vi "1B_BFG Ramp Data.vi"(7 "array":dbl[][](array[numeric])=array2400x3[7200 elements]) -> (8 "Threshold Values":u16[](array[numeric]))   [LabVIEW 2010]
panel:
  # "•\tBattery 75% Voltage Threshold, No Load: 3.950V\n•\tBattery 75% Voltage Threshold, Stimulation On: 3.925V\n•\tBattery 50% Voltage Threshold, No Load: 3.850V\n•\tBattery 50% Voltage Threshold, Stimulation On: 3.825V\n•\tBattery 25% Voltage Threshold, No Load: 3.780V\n•\tBattery 25% Voltage Threshold, Stimulation On: 3.755V\n•\tBattery Warning Voltage Threshold, No Load: 3.740V\n•\tBattery Warning Voltage Threshold, Stimulation On: 3.715V\n•\tBattery Critical Voltage Threshold, No Load: 3.720V\n•\tBattery Critical Voltage Threshold, Stimulation On: 3.695V\n•\tMinimum Safe Stimulating Voltage, No Load: 3.700V\n•\tMinimum Safe Stimulation Voltage, Stimulation On: 3.675V\n•\tBattery Cut-off Voltage Threshold:  2.850V"
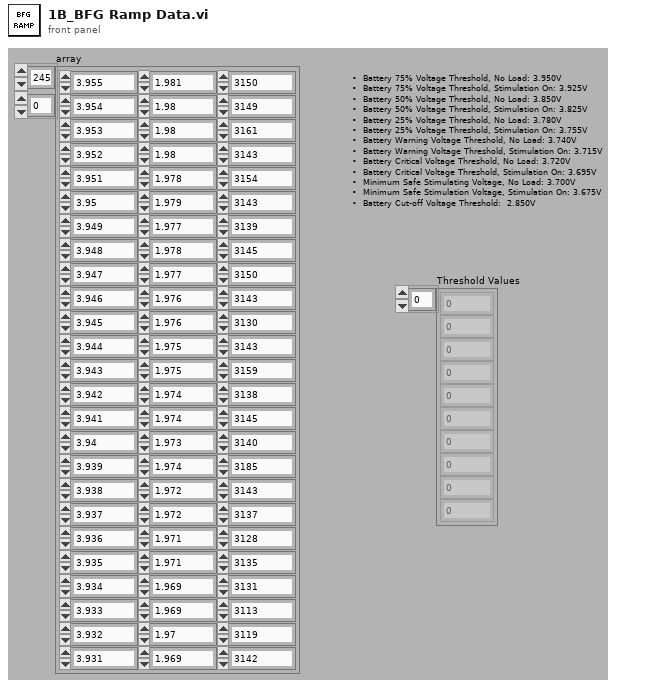
[diagram p1: front panel]
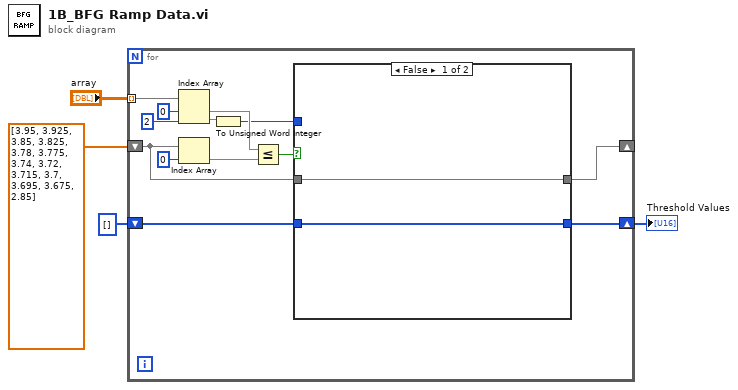
[diagram p0: block diagram]
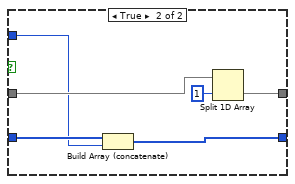
[diagram p2: hidden frame]
diagram:
  n1 = for {
    tunnel: "array" -> [w16] mode=indexing
    shift-right: [w6] -> _
    shift-left: dbl[] [3.95, 3.925, 3.85, 3.825, 3.78, 3.775, 3.74, 3.72, 3.715, 3.7, 3.695, 3.675, 2.85] -> [w7]
    shift-right: [w5] -> w1
    shift-left: u16[] [] -> [w8]
    n2 = Index Array(array=w16, index #1=0 ("index"), index #2=2 ("index")) -> (element #1=w12:dbl, element #2=w13:dbl)
    n3 = Index Array(array=w7, index=0) -> (element=w11:dbl)
    n4 = To Unsigned Word Integer(number=w13) -> (unsigned 16bit integer=w9:u16)
    n5 = Less Or Equal?(x=w12, y=w11) -> (x <= y?=w10:bool)
    n6 = case shown="False" w10 {
      tunnel: w9 -> [_ w20]
      tunnel: w8 -> [w18 w25]
      tunnel: w7 -> [w19 w24]
      tunnel: [w19 w23] -> w6
      tunnel: [w18 w21] -> w5
      frame False {
      }
      frame True {
        n7 = Build Array (concatenate)(w25, w20) -> (w21:u16[])
        n8 = Split 1D Array(array=w24, index=1) -> (second subarray=w23:dbl[])  [unwired: 1 out]
      }
    }
  }
  "Threshold Values" <- w1
